vi "FFT To Spectrum.vi"(0 "real FFT data":dbl[](array[numeric]), 5 "imaginary FFT data":dbl[](array[numeric]), 7 "spectrum type":enum8{"Power (Vrms^2)", "Amplitude (Vrms)"}(ring), 9 "sample rate (S/s)":dbl format="%#_6p", 11 "error in (no error)":errorcluster) -> (4 "spectrum out":dbl[](array[numeric]), 10 "df (Hz)":dbl, 15 "error out":errorcluster)   [LabVIEW 2017, in "NI_FpgaMspHost.lvlib"]
doc: "Converts the output of the Fast Fourier Transform (FFT) Express VI to a power or amplitude spectrum. The spectrum is single-sided and scaled."
uses:
  <vilib>/rvi/Analysis/host/Public/NI_FpgaMspHost.lvlib
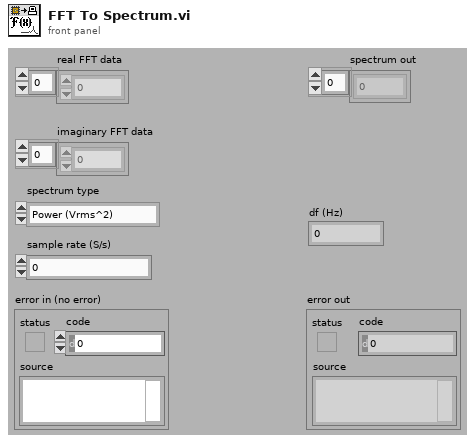
[diagram p1: front panel]
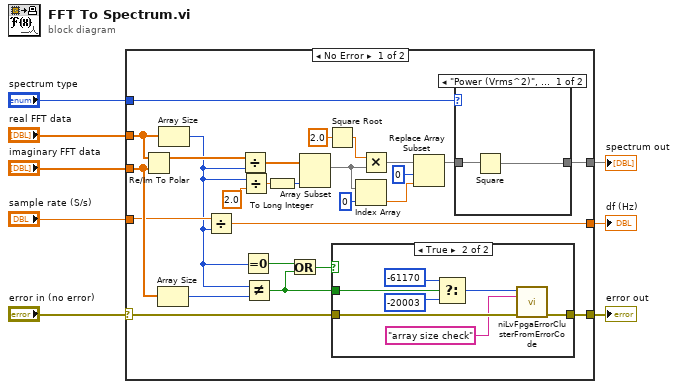
[diagram p0: block diagram]
diagram:
  n1 = case shown="No Error" "error in (no error)" {
    selector: "error in (no error)" -> [w14 w46]
    tunnel: "sample rate (S/s)" -> [w24 _]
    tunnel: [w13 w46] -> w7
    tunnel: "real FFT data" -> [w26 _]
    tunnel: "imaginary FFT data" -> [w25 _]
    tunnel: [w23 _] -> w3
    tunnel: "spectrum type" -> [w17 _]
    tunnel: [w15 _] -> w1
    frame No Error {
      n2 = Re/Im To Polar(2:w25, 3:w26) -> (1:w22:dbl[])  [unwired: 1 out]
      n3 = Array Size(array=w25) -> (size(s)=w20:i32)
      n4 = Array Size(array=w26) -> (size(s)=w12:i32)
      n5 = Divide(x=w24, y=w12) -> (x/y=w23:dbl)
      n6 = Divide(x=w22, y=w12) -> (x/y=w32:dbl[])
      n7 = Divide(x=w12, y=2.0) -> (x/y=w27:dbl)
      n8 = Equal To 0?(x=w12) -> (x = 0?=w11:bool)
      n9 = Not Equal?(x=w12, y=w20) -> (x != y?=w9:bool)
      n10 = To Long Integer(number=w27) -> (32bit integer=w19:i32)
      n11 = Or(x=w11, y=w9) -> (x .or. y?=w10:bool)
      n12 = Array Subset(array=w32, length=w19) -> (w29:dbl[])  [unwired: 1 in]
      n13 = Square Root(x=2.0) -> (sqrt(x)=w30:dbl)
      n14 = case shown="True" w10 {
        tunnel: [w35 w42] -> w13
        tunnel: w14 -> [w35 w41]
        tunnel: w9 -> [_ w37]
        frame False {
        }
        frame True {
          n15 = Select(t=-61170 ("error code"), s=w37, f=-20003 ("error code")) -> (s? t:f=w38:i32)
          n16 = call <vilib>:"niLvFpgaErrorClusterFromErrorCode.vi"("error code"=w38, "function name"="array size check" ("L10N_Function Name"), "error in"=w41) -> ("error out"=w42:errorcluster)  [unwired: 4 in, 8 out]
        }
      }
      n17 = Index Array(array=w29, index=0) -> (element=w18:dbl)
      n18 = Multiply(x=w30, y=w29) -> (x*y=w31:dbl[])
      n19 = Replace Array Subset(array=w31, new element=w18, index=0) -> (w16:dbl[])
      n20 = case shown="\"Power (Vrms^2)\", Default" w17 {
        tunnel: w16 -> [w44 w45]
        tunnel: [w43 w45] -> w15
        frame "Power (Vrms^2)", Default {
          n21 = Square(x=w44) -> (x^2=w43:dbl[])
        }
        frame "Amplitude (Vrms)" {
        }
      }
    }
    frame Error {
    }
  }
  "error out" <- w7
  "df (Hz)" <- w3
  "spectrum out" <- w1
